vi "Area_gadgets_triangulo.vi"() -> ()   [LabVIEW 2020]
panel:
  in  "ALTURA":dbl(slide) scale=0.0..30.0
  in  "BASE":dbl(slide) scale=0.0..30.0
  in  "Horizontal Pointer Slide":dbl(slide) scale=1.8..2.0
  out "Area del Triangulo":dbl(knob) scale=0.0..100.0
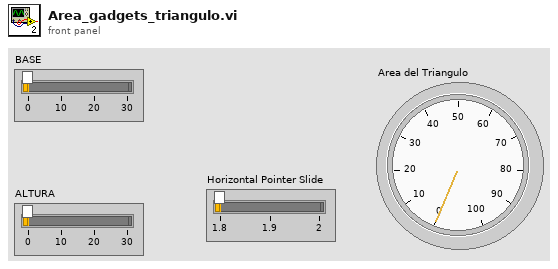
[diagram p1: front panel]
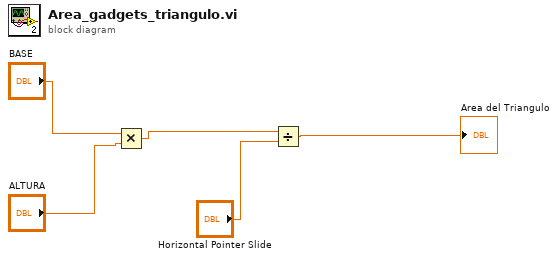
[diagram p0: block diagram]
diagram:
  n1 = Multiply(x="BASE", y="ALTURA") -> (x*y=w3:dbl)
  n2 = Divide(x=w3, y="Horizontal Pointer Slide") -> (x/y=→"Area del Triangulo":dbl)
